vi "datapathsubvi.vi"(10 "Data":enum16{"191122", "191123", "200410", ""}(ring), 11 "default data path":path) -> (3 "appended path":path)   [LabVIEW 2018, in "analysis.lvlib"]
uses:
  analysis.lvlib
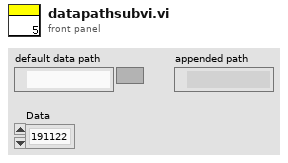
[diagram p1: front panel]
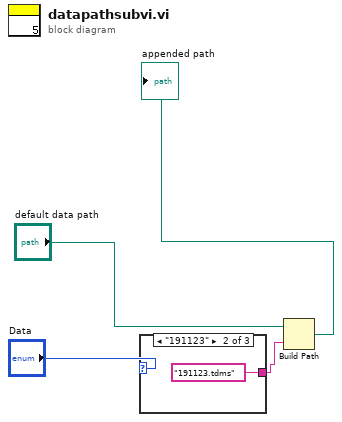
[diagram p0: block diagram]
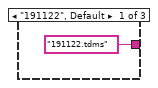
[diagram p2: hidden frame]
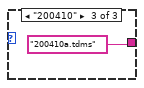
[diagram p3: hidden frame]
diagram:
  n1 = case shown="\"191123\"" "Data" {
    tunnel: ["191122.tdms" ("name or relative path") "191123.tdms" ("name or relative path") "200410a.tdms" ("name or relative path")] -> w3
    frame "191122", Default {
    }
    frame "191123" {
    }
    frame "200410" {
    }
  }
  n2 = Build Path(base path="default data path", name or relative path=w3) -> (appended path=→"appended path":path)
